vi "Fahenheit Readout Thing.vi"() -> ()   [LabVIEW 2018]
panel:
  out "Waveform Graph":dbl[](graph)
  out "Waveform Chart":dynamicdata(graph)
  out "Numeric":dbl
  in  "Slide":dbl(slide) scale=0.0..50.0
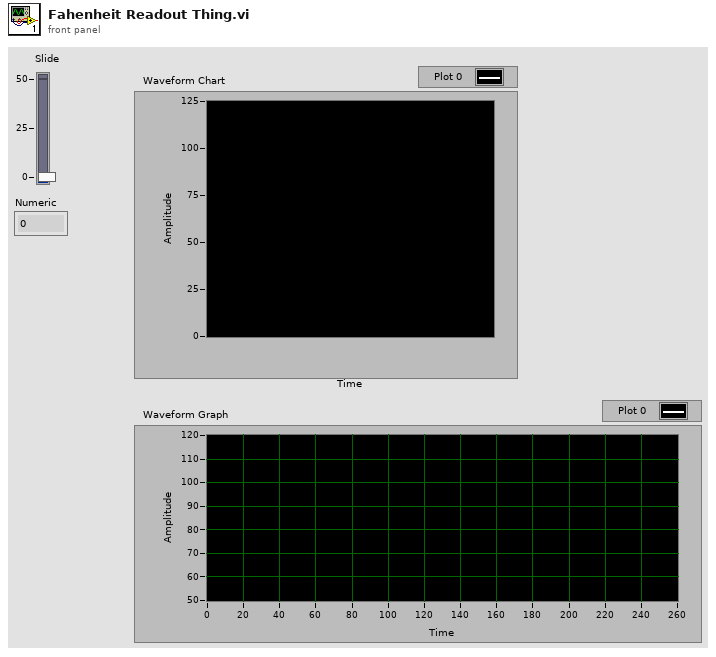
[diagram p1: front panel]
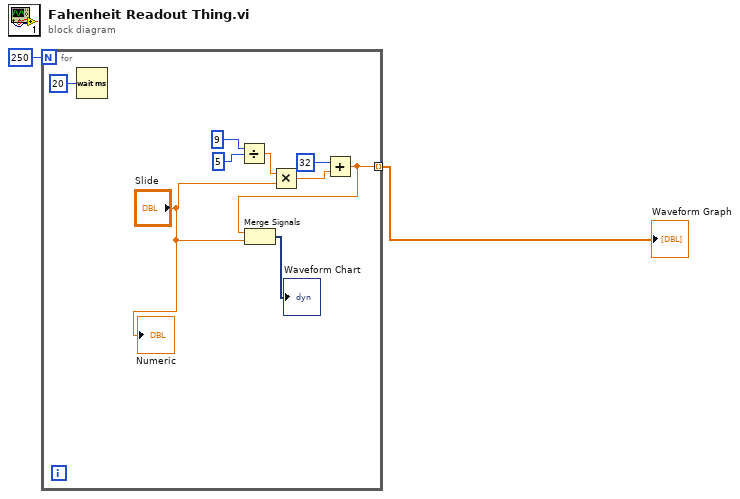
[diagram p0: block diagram]
diagram:
  n1 = for {
    N: 250 -> [_]
    tunnel: [w3] -> w1 mode=indexing
    n2 = Wait (ms)(milliseconds to wait=u32 20) -> ()  [unwired: 1 out]
    n3 = Divide(x=9, y=5) -> (x/y=w9:dbl)
    n4 = Multiply(x=w9, y="Slide") -> (x*y=w7:dbl)
    n5 = Add(x=32, y=w7) -> (x+y=w3:dbl)
    n6 = Merge Signals(w3, "Slide") -> (→"Waveform Chart":dynamicdata)
    "Numeric" <- "Slide"
  }
  "Waveform Graph" <- w1
